vi "Init_core.vi"(8 "error in (no error)":errorcluster, 10 "VIRefIn":refnum<vi>, 11 "ctlRef_Maps in":refnum<class "ctlRef_Maps.lvclass">) -> (0 "error out":errorcluster, 3 "ctlRef_Maps out":refnum<class "ctlRef_Maps.lvclass">)   [LabVIEW 2020, in "CtlReferences.lvlib" / "ctlRef_Maps.lvclass"]
uses:
  ctlRef_Maps.lvclass
  ctlRef_Maps.lvclass/ctlRef_Maps.ctl
  CtlReferences/CtlReferences.lvclass
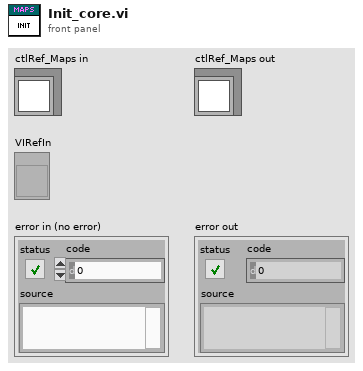
[diagram p1: front panel]
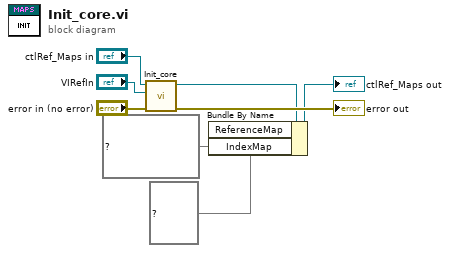
[diagram p0: block diagram]
diagram:
  n1 = call-parent "Init_core.vi"("error in (no error)"="error in (no error)", "VIRefIn"="VIRefIn", "CtlReferences in"="ctlRef_Maps in") -> ("error out"=→"error out":errorcluster, "CtlReferences out"=w7:refnum<class "ctlRef_Maps.lvclass">)  [unwired: 7 in]
  n2 = Bundle By Name(cluster=w7, "ReferenceMap"=map{string, refnum<vi>} {}, "IndexMap"=map{string, i32} {}) -> (→"ctlRef_Maps out":refnum<class "ctlRef_Maps.lvclass">)
